vi "niTuner Set Freq(spec array).vi"(8 "error in":errorcluster, 10 "desired RF spectra":T3(array[cluster]) {"resolution bandwidth" format="%.2p"; "RF frequency" format="%.2p"; "span" format="%.2p"}, 11 "taskID in":i32 format="%.0x") -> (0 "error out":errorcluster, 1 "actual RF tuned spectra":T1(array[cluster]) {"resolution bandwidth" format="%.2p"; "RF tuned frequency" format="%.2p"; "span" format="%.2p"}, 2 "actual IF spectra":T2(array[cluster]) {"resolution bandwidth" format="%.2p"; "IF frequency" format="%.2p"; "span" format="%.2p"}, 3 "taskID out":i32 format="%.0x", 4 "frequency shifts":dbl[](array[numeric]) format="%.2p")   [LabVIEW 2011]
doc: "This polymorph sets up to 720 spectra with center frequencies in the scan list. The PXI-5600 downconverter does not go to the first frequency until niTuner Initiate Scan.vi is called. When triggered, the PXI-5600 downconverter tunes to the scan list entries in succession. The format of the \"spectrum settings\" inputs and outputs is designed to provide a convenient interface with the Spectral Measurements Toolset (SMT).\n\nNOTE: If new center frequencies of less than 15 MHz are specified by a call to this VI, attenuation may be automatically adjusted. Up to 20 dB additional attenuation may be added."
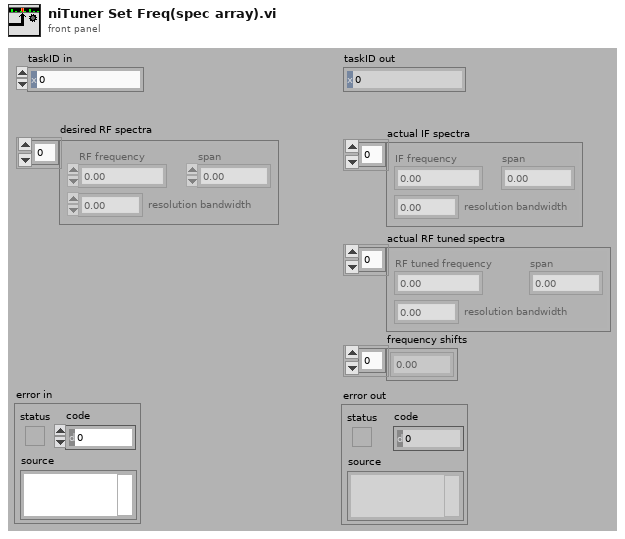
[diagram p1: front panel]
types:
  T1 = cluster{"RF tuned frequency":dbl, "span":dbl, "resolution bandwidth":dbl}[]
  T2 = cluster{"IF frequency":dbl, "span":dbl, "resolution bandwidth":dbl}[]
  T3 = cluster{"RF frequency":dbl, "span":dbl, "resolution bandwidth":dbl}[]
  T4 = cluster{"RF frequency":dbl, "span":dbl, "resolution bandwidth":dbl}
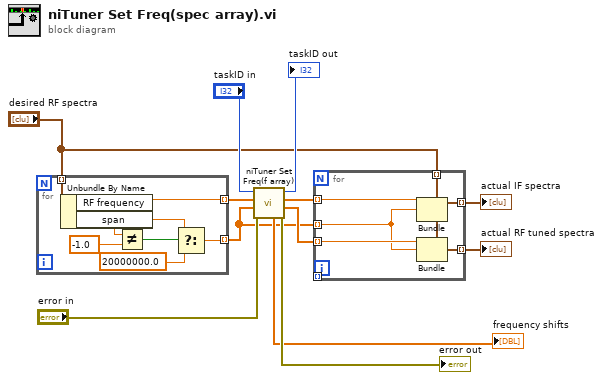
[diagram p0: block diagram]
diagram:
  n1 = for {
    tunnel: "desired RF spectra" -> [w19] mode=indexing
    tunnel: [w14] -> w6 mode=indexing
    tunnel: [w13] -> w1 mode=indexing
    n2 = Unbundle By Name(w19) -> ("RF frequency"=w14:dbl, "span"=w18:dbl)
    n3 = Not Equal?(x=w18, y=-1.0) -> (x != y?=w16:bool)
    n4 = Select(t=w18, s=w16, f=20000000.0) -> (s? t:f=w13:dbl)
  }
  n5 = call <instrlib>:"niTuner Set Freq(f array).vi"("error in"="error in", "spans"=w1, "desired RF frequencies"=w6, "taskID in"="taskID in") -> ("error out"=→"error out":errorcluster, "actual RF tuned frequencies"=w4:dbl[], "actual IF frequencies"=w5:dbl[], "taskID out"=→"taskID out":i32, "frequency shifts"=→"frequency shifts":dbl[])  [unwired: 3 in]
  n6 = for {
    tunnel: w5 -> [w26] mode=indexing
    tunnel: w4 -> [w25] mode=indexing
    tunnel: [w24] -> w9 mode=indexing
    tunnel: [w23] -> w8 mode=indexing
    tunnel: [w22] -> _ mode=indexing
    tunnel: "desired RF spectra" -> [w21] mode=indexing
    tunnel: w1 -> [w20] mode=indexing
    i -> [w22]
    n7 = Bundle(cluster=w21, "RF frequency"=w26, "span"=w20) -> (w24:T4)  [unwired: 1 in]
    n8 = Bundle(cluster=w21, "RF frequency"=w25, "span"=w20) -> (w23:T4)  [unwired: 1 in]
  }
  "actual IF spectra" <- w9
  "actual RF tuned spectra" <- w8
